vi "VF Laser Control.vi"(0 "Laser Notifier Element":T1={"Laser Action"=enum."Set On/Off", "Received?"=FALSE, "Enabled (Interlock)?"=FALSE, "Light Emission?"=FALSE, "Power (mW)"=0.0, "Settings"={"Laser Parameters"=enum."Wavelength (nm)", "Value"=0.0}, "Status"=enum."Error", "Error"={"status"=FALSE, "code"=0, "source"=""}}, 11 "VISA Ref":refnum<visa-resource-name>) -> (4 "Laser Notifier Element":T1={"Laser Action"=enum."Set On/Off", "Received?"=FALSE, "Enabled (Interlock)?"=FALSE, "Light Emission?"=FALSE, "Power (mW)"=0.0, "Settings"={"Laser Parameters"=enum."Wavelength (nm)", "Value"=0.0}, "Status"=enum."Error", "Error"={"status"=FALSE, "code"=0, "source"=""}})   [LabVIEW 2020]
uses:
  Laser Controls/Laser Notifier Element.ctl
  Laser Controls/Laser Actions.ctl
  Laser Controls/Laser Settings.ctl
  Laser Controls/Laser Parameters.ctl
  Laser Controls/Laser Status.ctl
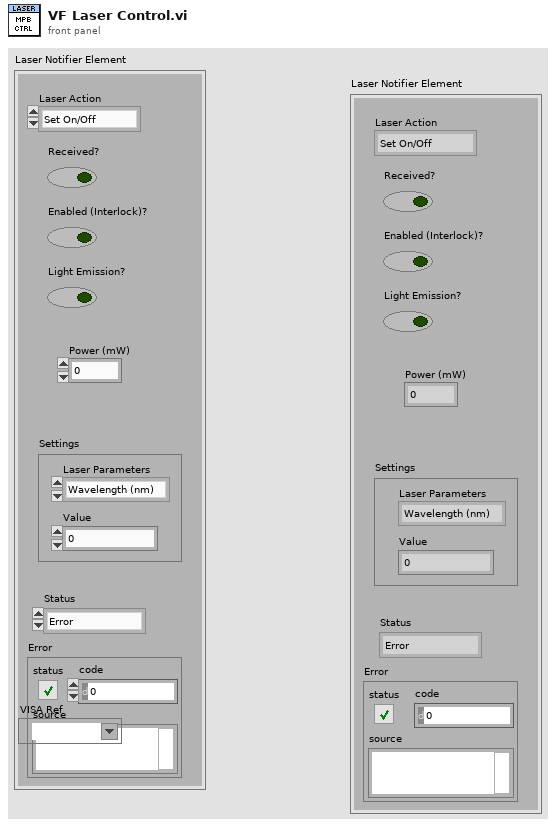
[diagram p1: front panel]
types:
  T1 = typedef "Laser Notifier Element.ctl" = cluster{"Laser Action":T2, "Received?":bool, "Enabled (Interlock)?":bool, "Light Emission?":bool, "Power (mW)":dbl, "Settings":T3, "Status":T5, "Error":errorcluster}
  T2 = typedef "Laser Actions.ctl" = enum16{"Error Check", "Set On/Off", "Set Power", "Set Parameter", "Get Power", "Get Status", "Get Parameter", "Quit"}
  T3 = typedef "Laser Settings.ctl" = cluster{"Laser Parameters":T4, "Value":dbl}
  T4 = typedef "Laser Parameters.ctl" = enum16{"Wavelength (nm)", "Pulsing?", "Rep. Rate", "External Control"}
  T5 = typedef "Laser Status.ctl" = enum16{"Warmup", "Ready", "Emission", "Tuning", "Error"}
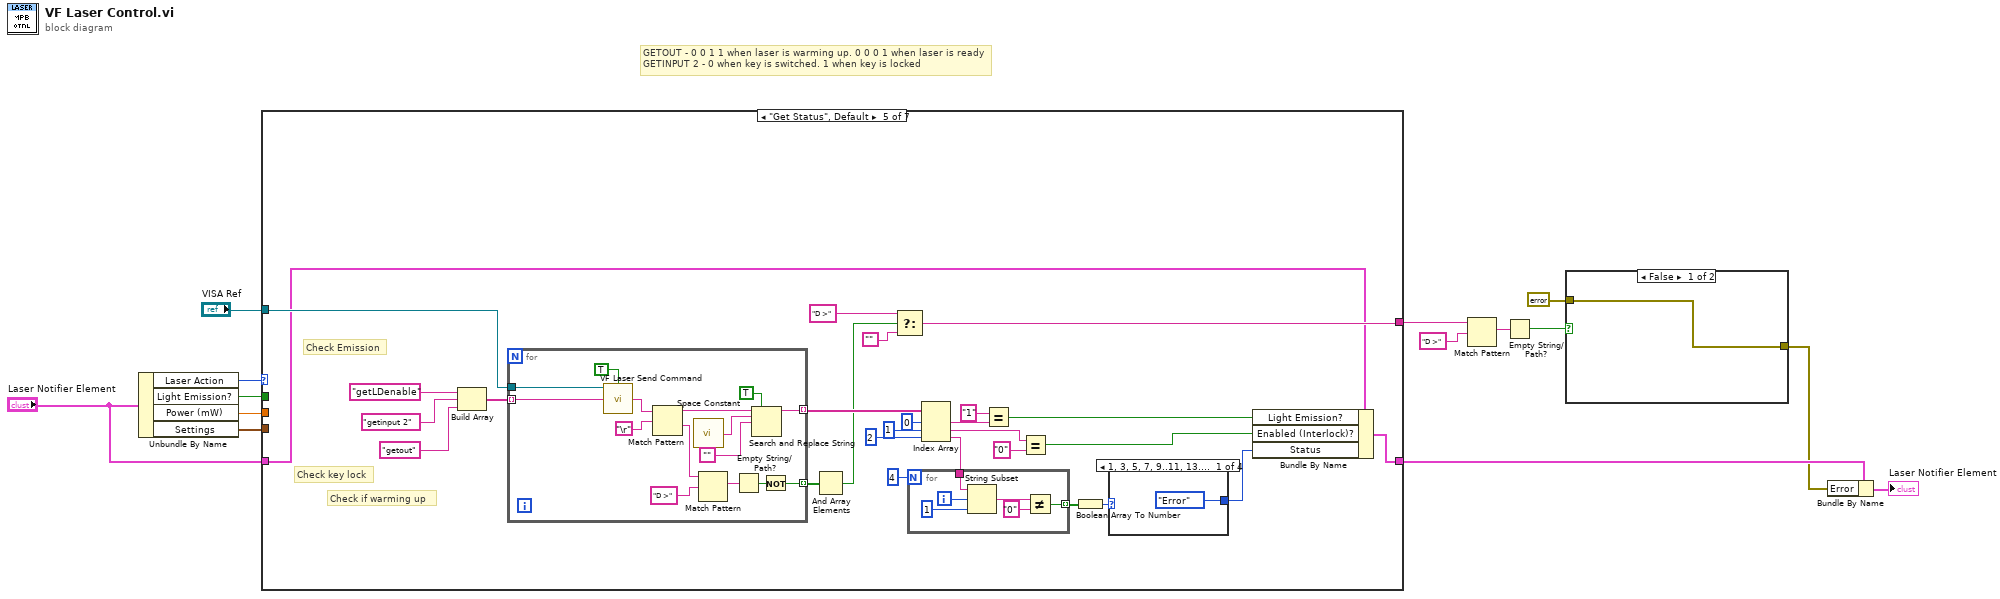
[diagram p0: block diagram]
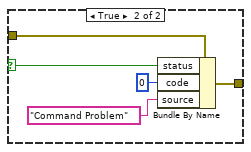
[diagram p2: hidden frame]
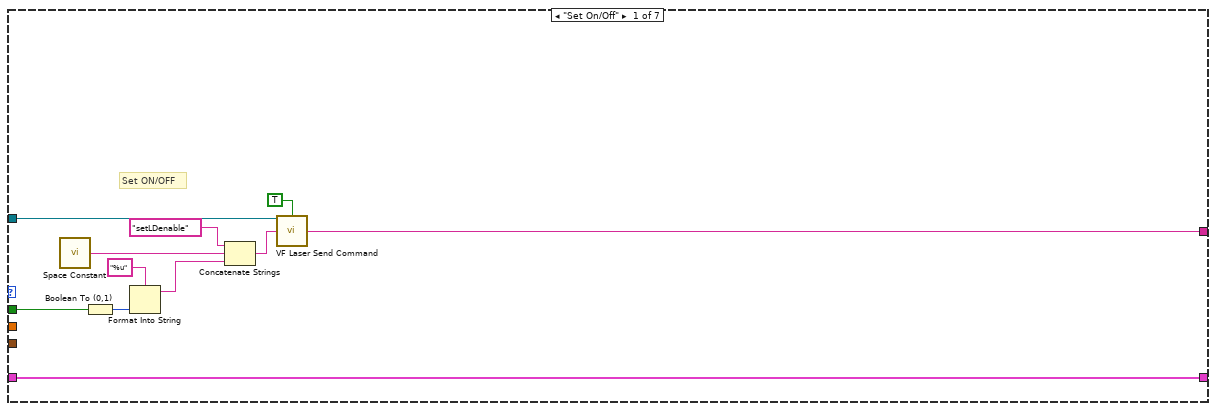
[diagram p3: hidden frame]
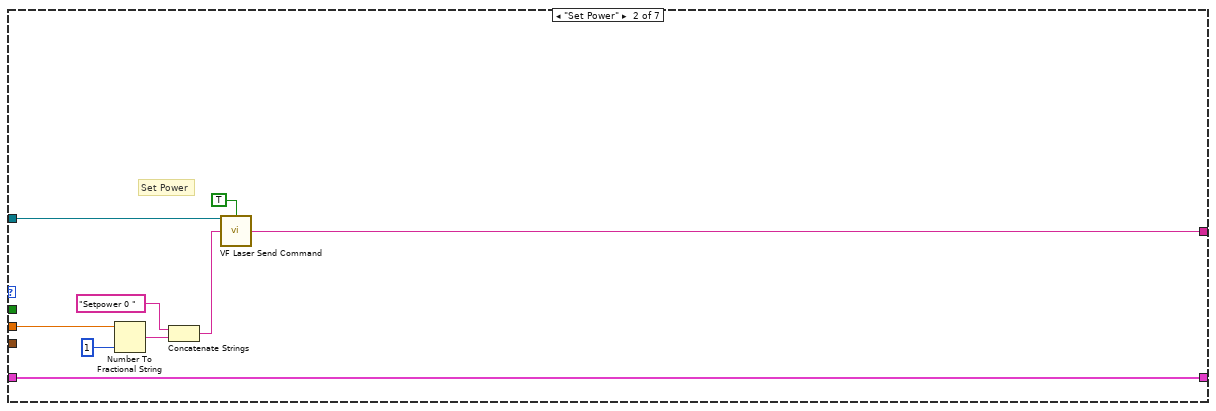
[diagram p4: hidden frame]
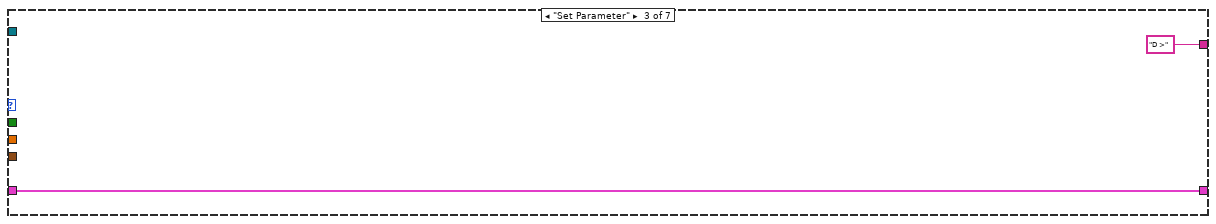
[diagram p5: hidden frame]
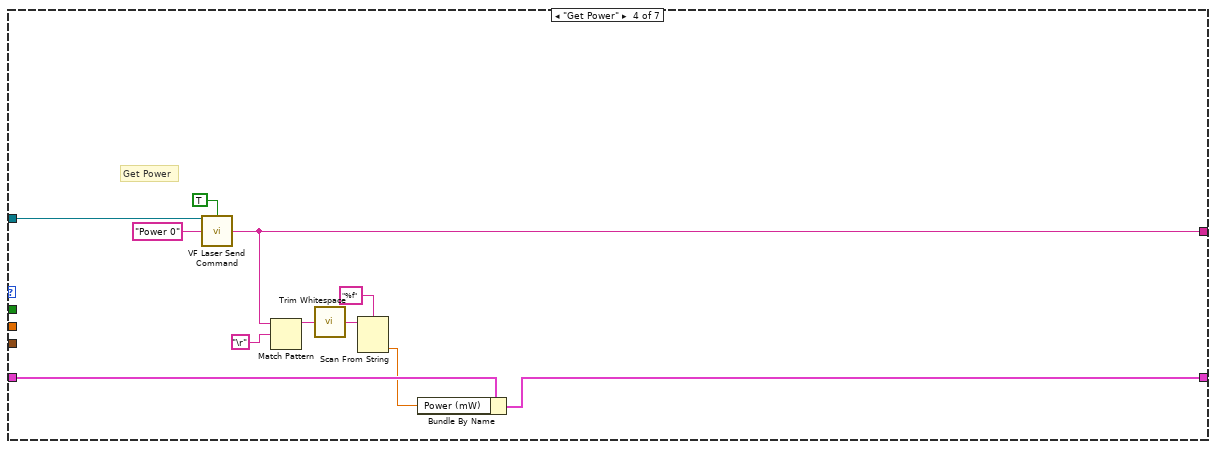
[diagram p6: hidden frame]
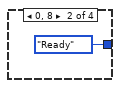
[diagram p7: hidden frame]
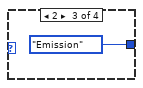
[diagram p8: hidden frame]
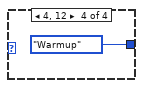
[diagram p9: hidden frame]
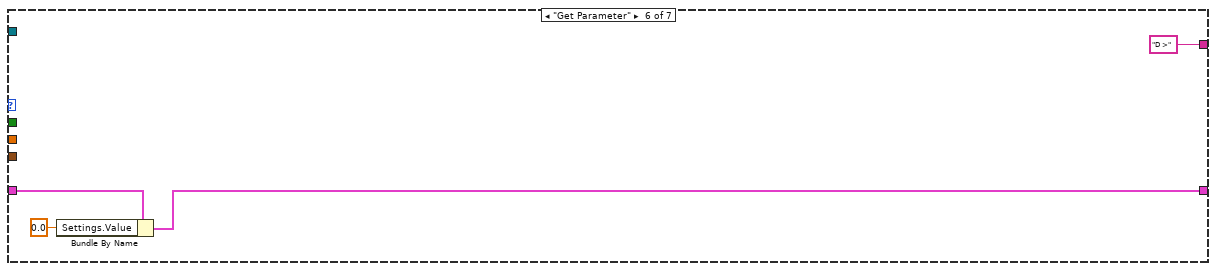
[diagram p10: hidden frame]
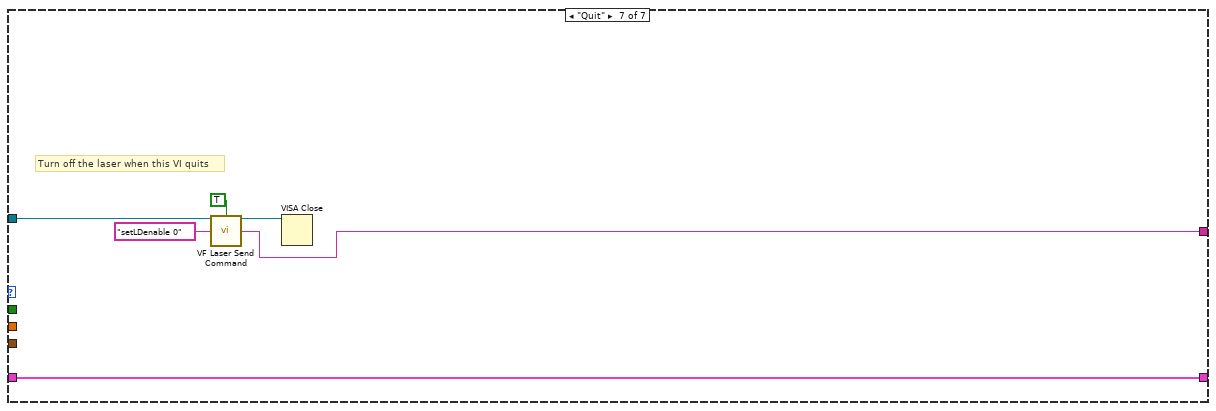
[diagram p11: hidden frame]
diagram:
  # "GETOUT - 0 0 1 1 when laser is warming up. 0 0 0 1 when laser is ready\nGETINPUT 2 - 0 when key is switched. 1 when key is locked"
  n1 = Unbundle By Name("Laser Notifier Element") -> ("Laser Action"=w14:T2, "Light Emission?"=w5:bool, "Power (mW)"=w4:dbl, "Settings"=w3:T3)
  n2 = case shown="\"Get Status\", Default" w14 {
    tunnel: "VISA Ref" -> [w19 w30 _ w42 w72 _ w107]
    tunnel: [w15 w26 "D >" ("Response") w37 w60 "D >" ("Response") w104] -> w1
    tunnel: [w17 w28 w36 w39 w71 w101 w106] -> w8
    tunnel: w5 -> [w18 _ _ _ _ _ _]
    tunnel: w4 -> [_ w29 _ _ _ _ _]
    tunnel: w3 -> [_ _ _ _ _ _ _]
    tunnel: "Laser Notifier Element" -> [w17 w28 w36 w41 w48 w103 w106]
    frame "Set On/Off" {
      # "Set ON/OFF"
      n3 = call <vilib>:"Space Constant.vi"() -> ("String"=w21:string)
      n4 = Boolean To (0,1)(Boolean=w18) -> (0, 1=w20:i16)
      n5 = Format Into String(format string="%u", w20) -> (resulting string=w23:string)  [unwired: 2 in, 1 out]
      n6 = Concatenate Strings("setLDenable" ("string"), w21, w23) -> (w16:string)
      n7 = call "VF Laser Send Command.vi"("VISA Ref"=w19, "Wait for Reply (T)"=TRUE ("Wait for Reply?"), "Command"=w16) -> ("Reply"=w15:string)  [unwired: 10 in, 2 out]
    }
    frame "Set Power" {
      # "Set Power"
      n8 = Number To Fractional String(number=w29, precision (6)=i16 1) -> (F-format string=w34:string)  [unwired: 2 in]
      n9 = Concatenate Strings("Setpower 0 " ("string"), w34) -> (w27:string)
      n10 = call "VF Laser Send Command.vi"("VISA Ref"=w30, "Wait for Reply (T)"=TRUE ("Wait for Reply?"), "Command"=w27) -> ("Reply"=w26:string)  [unwired: 10 in, 2 out]
    }
    frame "Set Parameter" {
    }
    frame "Get Power" {
      # "Get Power"
      n11 = call "VF Laser Send Command.vi"("VISA Ref"=w42, "Wait for Reply (T)"=TRUE ("Wait for Reply?"), "Command"="Power 0" ("string")) -> ("Reply"=w37:string)  [unwired: 10 in, 2 out]
      n12 = Match Pattern(string=w37, regular expression="\r") -> (before substring=w43:string)  [unwired: 1 in, 3 out]
      n13 = call <vilib>:"Trim Whitespace.vi"("string"=w43) -> ("trimmed string"=w45:string)  [unwired: 1 in]
      n14 = Scan From String(format string="%f", input string=w45) -> (output 1=w40:dbl)  [unwired: 3 in, 3 out]
      n15 = Bundle By Name(cluster=w41, "Power (mW)"=w40) -> (w39:T1)
    }
    frame "Get Status", Default {
      # "Check Emission"
      # "Check key lock"
      # "Check if warming up"
      n16 = Build Array("getLDenable" ("string"), "getinput 2" ("string"), "getout" ("string")) -> (w74:string[])
      n17 = for {
        tunnel: w74 -> [w86] mode=indexing
        tunnel: [w87] -> w68 mode=indexing
        tunnel: w72 -> [w98]
        tunnel: [w92] -> w64 mode=indexing
        n18 = call "VF Laser Send Command.vi"("VISA Ref"=w98, "Wait for Reply (T)"=TRUE ("Wait for Reply?"), "Command"=w86) -> ("Reply"=w85:string)  [unwired: 10 in, 2 out]
        n19 = Match Pattern(string=w85, regular expression="\r") -> (before substring=w88:string, after substring=w94:string)  [unwired: 1 in, 2 out]
        n20 = call <vilib>:"Space Constant.vi"() -> ("String"=w90:string)
        n21 = Match Pattern(string=w94, regular expression="D >" ("Response")) -> (match substring=w96:string)  [unwired: 1 in, 3 out]
        n22 = Empty String/Path?(string/path=w96) -> (empty?=w93:bool)
        n23 = Search and Replace String(replace all?=TRUE ("replace all? (F)"), input string=w88, search string=w90, replace string="") -> (result string=w87:string)  [unwired: 4 in, 3 out]
        n24 = Not(x=w93) -> (.not. x?=w92:bool)
      }
      n25 = And Array Elements(Boolean array=w64) -> (logical AND=w63:bool)
      n26 = Select(t="D >" ("Response"), s=w63, f="") -> (s? t:f=w60:string)
      n27 = Index Array(array=w68, index #1=0 ("index"), index #2=1 ("index"), index #3=2 ("index")) -> (element #1=w59:string, element #2=w54:string, element #3=w53:string)
      n28 = for {
        N: 4 -> [_]
        tunnel: [w80] -> w51 mode=indexing
        tunnel: w53 -> [w79]
        i -> [w83]
        n29 = String Subset(string=w79, offset (0)=w83, length (rest)=1 ("length (rest)")) -> (substring=w82:string)
        n30 = Not Equal?(x=w82, y="0") -> (x != y?=w80:bool)
      }
      n31 = Equal?(x="1", y=w59) -> (x = y?=w57:bool)
      n32 = Equal?(x=w54, y="0" ("x")) -> (x = y?=w55:bool)
      n33 = Boolean Array To Number(Boolean array=w51) -> (number=w50:u32)
      n34 = case shown="1, 3, 5, 7, 9..11, 13..15, Default" w50 {
        tunnel: [Laser_Status."Error" ("Status") Laser_Status."Ready" ("Status") Laser_Status."Emission" ("Status") Laser_Status."Warmup" ("Status")] -> w49
        frame 1, 3, 5, 7, 9..11, 13..15, Default {
        }
        frame 0, 8 {
        }
        frame 2 {
        }
        frame 4, 12 {
        }
      }
      n35 = Bundle By Name(cluster=w48, "Light Emission?"=w57, "Enabled (Interlock)?"=w55, "Status"=w49) -> (w71:T1)
    }
    frame "Get Parameter" {
      n36 = Bundle By Name(cluster=w103, "Settings.Value"=0.0) -> (w101:T1)
    }
    frame "Quit" {
      # "Turn off the laser when this VI quits"
      n37 = call "VF Laser Send Command.vi"("VISA Ref"=w107, "Wait for Reply (T)"=TRUE ("Wait for Reply?"), "Command"="setLDenable 0" ("string")) -> ("VISA Ref Dup"=w108:refnum<visa-resource-name>, "Reply"=w104:string)  [unwired: 10 in, 1 out]
      n38 = VISA Close(VISA resource name=w108) -> ()  [unwired: 1 in, 1 out]
    }
  }
  n39 = Match Pattern(string=w1, regular expression="D >" ("Response")) -> (match substring=w11:string)  [unwired: 1 in, 3 out]
  n40 = Empty String/Path?(string/path=w11) -> (empty?=w10:bool)
  n41 = case shown="False" w10 {
    selector: w10 -> [_ w112]
    tunnel: errorcluster {"status"=FALSE, "code"=0, "source"=""} ("Error") -> [w110 w113]
    tunnel: [w110 w111] -> w6
    frame False {
    }
    frame True {
      n42 = Bundle By Name(cluster=w113, "status"=w112, "code"=0, "source"="Command Problem") -> (w111:errorcluster)
    }
  }
  n43 = Bundle By Name(cluster=w8, "Error"=w6) -> (→"Laser Notifier Element":T1)
